vi "EventsRobotStuck.vi"(0 "our_robots":T3[](array[typedef]), 2 "Our_Robots frame":T1[](array[typedef]) {"height" format="%+4.3f"; "pixel_y" format="%+4.3f"; "pixel_x" format="%+4.3f"; "orientation" format="%+4.3f"; "y" format="%+4.3f"; "confidence" format="%4.3f"; "x" format="%+4.3f"}, 4 "FPS":dbl) -> (8 "Array":cluster{"ID":i32, "Relative error":dbl}[](array[cluster]))   [LabVIEW 2017]
uses:
  Core/AI Robot.ctl
  Intel/Functions Enum.ctl
  Intel/AttackerStates.ctl
  Path Planning/RRT/PathDests.ctl
  Path Planning/RRT/PathDest.ctl
  SSL Detection Robot.ctl
  <vilib>/Analysis/Matrix/Datatypes/RealMatrix.ctl
  <vilib>/Analysis/Matrix/NI_Matrix.lvlib
panel:
  out "Robot Stuck":bool
  out "empty?":bool
  out "Boolean":bool=TRUE
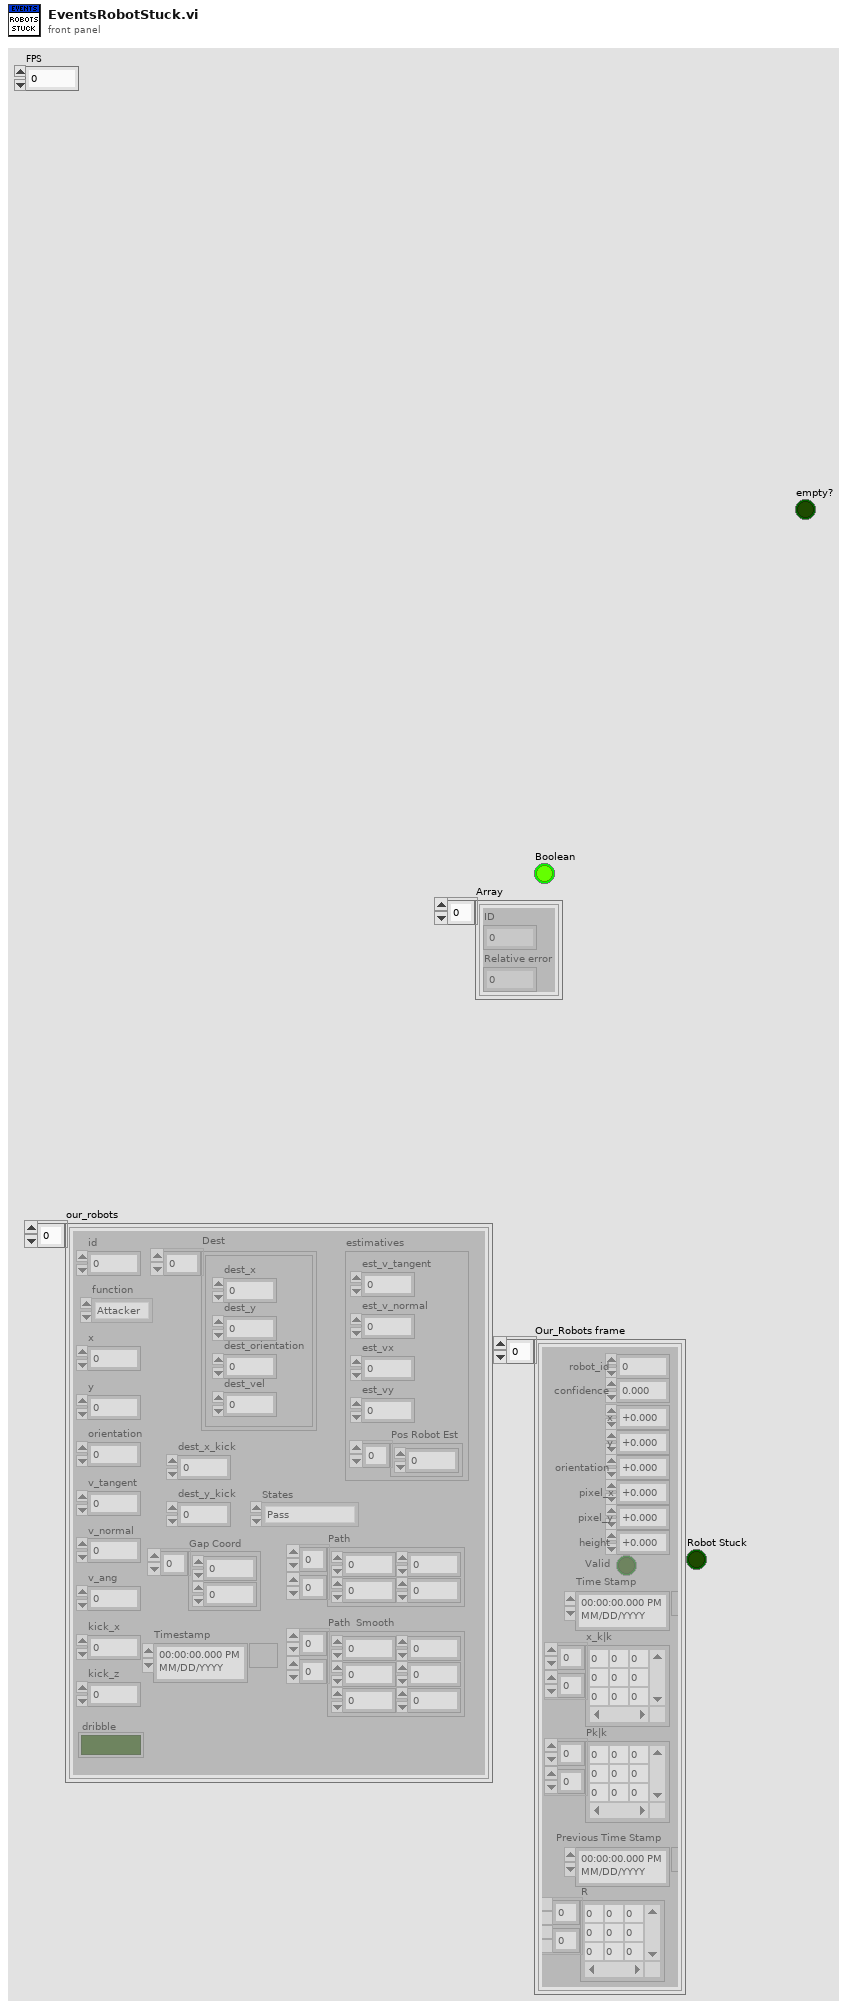
[diagram p1: front panel]
types:
  T1 = typedef "SSL Detection Robot.ctl" = cluster{"x":sgl, "robot_id":u32, "confidence":sgl, "y":sgl, "orientation":sgl, "pixel_x":sgl, "pixel_y":sgl, "height":sgl, "Valid":bool, "Time Stamp":timestamp, "x_k|k":T2, "Pk|k":T2, "Previous Time Stamp":timestamp, "R":T2}
  T2 = typedef "NI_Matrix.lvlib/RealMatrix.ctl" = dbl[][]
  T3 = typedef "AI Robot.ctl" = cluster{"id":u32, "function":T4, "x":dbl, "y":dbl, "orientation":dbl, "v_tangent":dbl, "v_normal":dbl, "v_ang":dbl, "kick_x":dbl, "kick_z":dbl, "dribble":bool, "Timestamp":timestamp, "estimatives":cluster{"est_v_tangent":dbl, "est_v_normal":dbl, "est_vx":dbl, "est_vy":dbl, "Pos Robot Est":dbl[]}, "dest_x_kick":dbl, "dest_y_kick":dbl, "Gap Coord":dbl[], "States":T5, "Path ":dbl[][], "Path  Smooth":dbl[][], "Dest":T6}
  T4 = typedef "Functions Enum.ctl" = enum16{"Attacker", "Goalie", "Defender", "Striker", "Goto 0", "Dummy", "Kicker", "ZigZag"}
  T5 = typedef "AttackerStates.ctl" = enum16{"Pass", "GoToTangent", "BallGetting", "GoToKick", ""}
  T6 = typedef "PathDests.ctl" = T7[]
  T7 = typedef "PathDest.ctl" = cluster{"dest_x":dbl, "dest_y":dbl, "dest_orientation":dbl, "dest_vel":dbl}
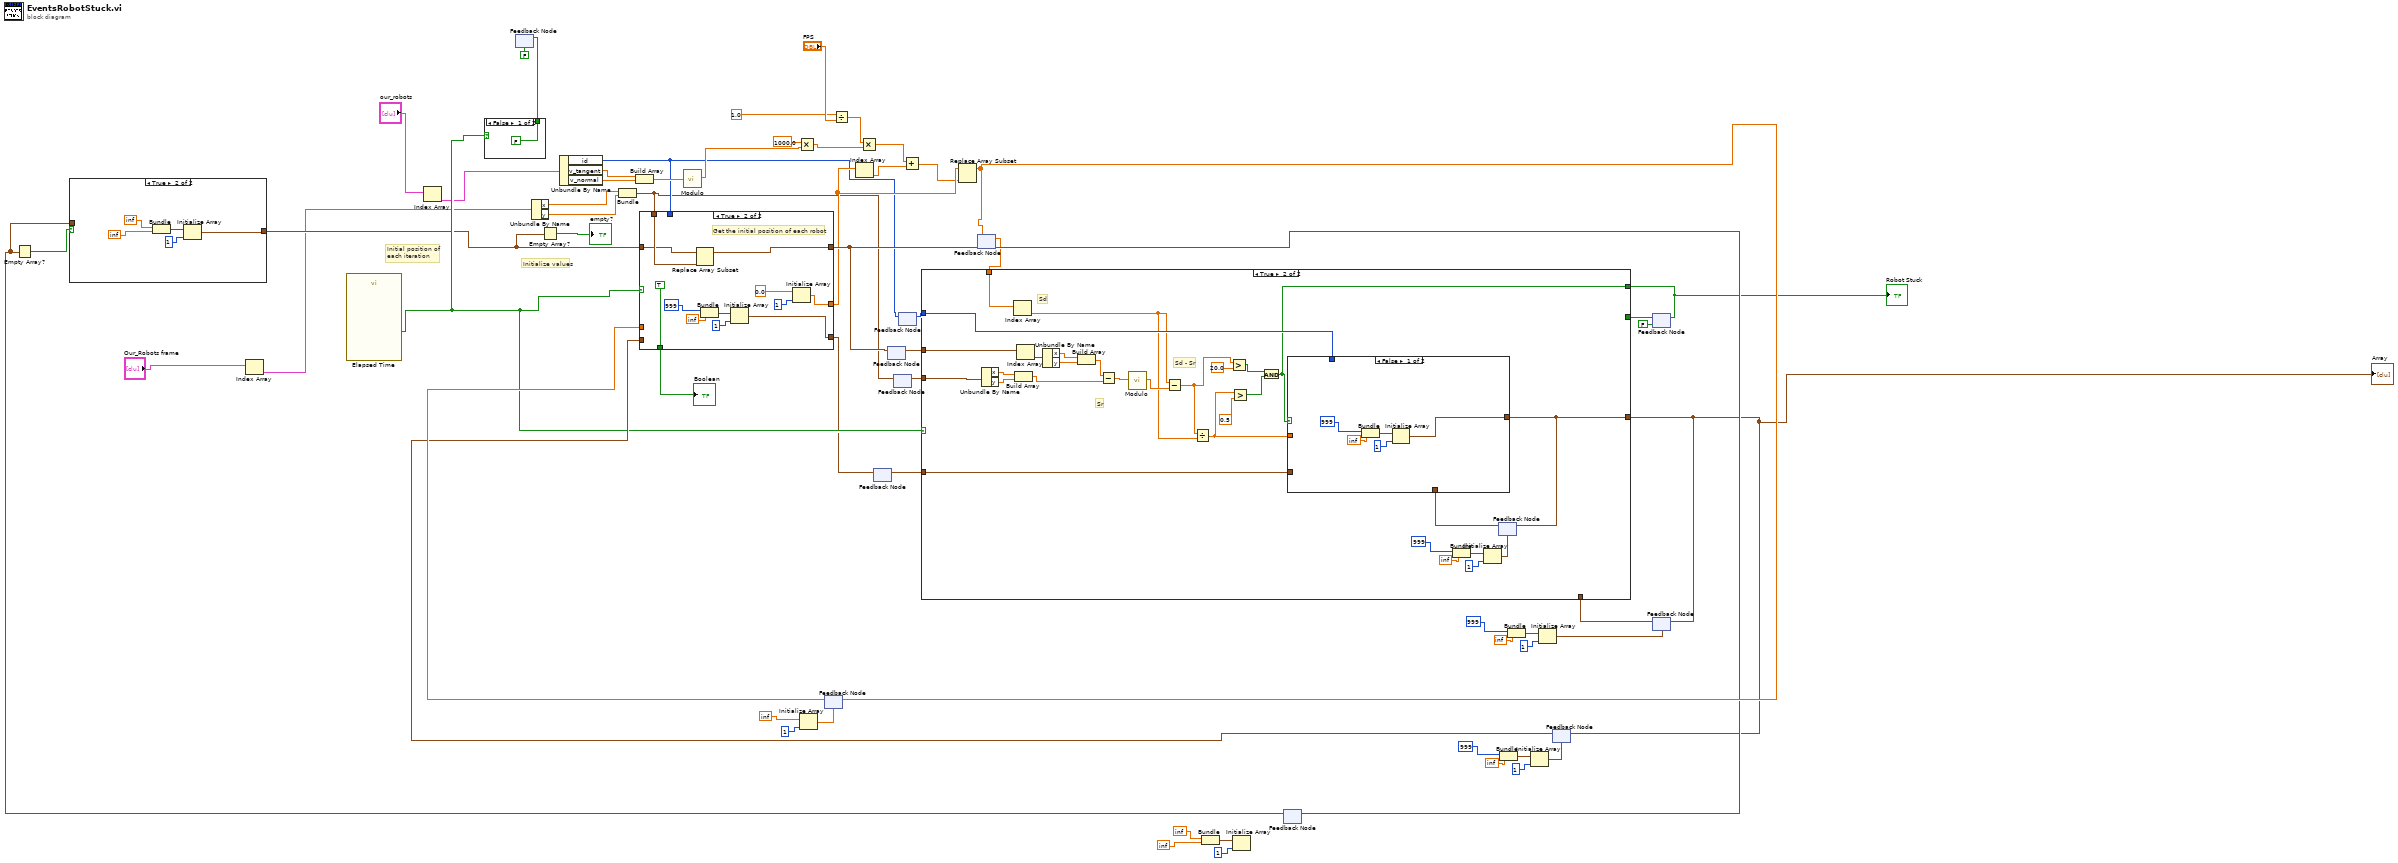
[diagram p0: block diagram]
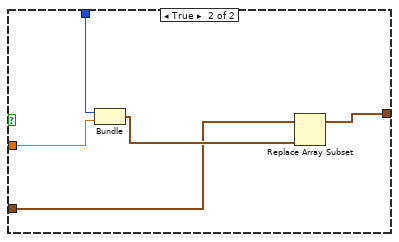
[diagram p3: hidden frame]
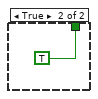
[diagram p4: hidden frame]
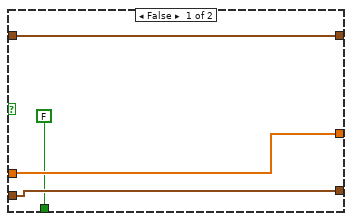
[diagram p5: hidden frame]
diagram:
  # "Initialize values"
  # "Initial position of\neach iteration"
  n1 = Index Array(array="Our_Robots frame") -> (element=w6:T1)  [unwired: 1 in]
  n2 = call "Elapsed Time"() -> ("Time has Elapsed"=w42:bool)  [unwired: 12 in, 7 out]
  n3 = Index Array(array="our_robots") -> (element=w3:T3)  [unwired: 1 in]
  n4 = case shown="False" w42 {
    tunnel: [FALSE TRUE] -> w50
    frame False {
    }
    frame True {
    }
  }
  n5 = feedback #1(FALSE) -> ()  [unwired: 1 in]
  n6 = feedback-in #1(w50) -> ()
  n7 = Unbundle By Name(w6) -> ("x"=w29:sgl, "y"=w28:sgl)
  n8 = Unbundle By Name(w3) -> ("id"=w11:u32, "v_tangent"=w38:dbl, "v_normal"=w37:dbl)
  n9 = Bundle("x"=w29, "y"=w28) -> (w8:cluster{"x":sgl, "y":sgl})  [unwired: 1 in]
  n10 = Build Array(w38, w37) -> (w36:dbl[])
  n11 = call "Modulo.vi"("2D vector"=w36) -> ("Modulo"=w27:dbl)  [unwired: 10 in]
  n12 = Multiply(x=1000.0, y=w27) -> (x*y=w25:dbl)
  n13 = Initialize Array(inf ("y"), 1 ("dimension size")) -> (w51:dbl[])
  n14 = feedback #2(w51) -> (w59:dbl[])
  n15 = Divide(x=1.0, y="FPS") -> (x/y=w33:dbl)
  n16 = Multiply(x=w33, y=w25) -> (x*y=w32:dbl)
  n17 = feedback #3() -> (w13:cluster{"ID":i32, "Relative error":dbl}[])  [unwired: 1 in]
  n18 = feedback #4() -> (w12:cluster{"x":sgl, "y":sgl}[])  [unwired: 1 in]
  n19 = feedback #5() -> (w7:cluster{"x":sgl, "y":sgl})  [unwired: 1 in]
  n20 = feedback-in #5(w8) -> ()
  n21 = feedback #6() -> (w10:u32)  [unwired: 1 in]
  n22 = feedback-in #6(w11) -> ()
  n23 = feedback #7() -> (w9:dbl[])  [unwired: 1 in]
  n24 = Bundle("x"=sgl inf, "y"=sgl inf) -> (w45:cluster{"x":sgl, "y":sgl})  [unwired: 1 in]
  n25 = Initialize Array(w45, 1 ("dimension size")) -> ()  [unwired: 1 out]
  n26 = feedback #8() -> (w39:cluster{"x":sgl, "y":sgl}[])  [unwired: 1 in]
  n27 = Empty Array?(array=w39) -> (empty?=w40:bool)
  n28 = case shown="True" w40 {
    tunnel: [w64 w65] -> w41
    tunnel: w39 -> [w64 _]
    frame False {
    }
    frame True {
      n29 = Bundle("x"=sgl inf, "y"=sgl inf) -> (w69:cluster{"x":sgl, "y":sgl})  [unwired: 1 in]
      n30 = Initialize Array(w69, 1 ("dimension size")) -> (w65:cluster{"x":sgl, "y":sgl}[])
    }
  }
  n31 = Empty Array?(array=w41) -> (empty?=→"empty?":bool)
  n32 = Bundle("dimension size"=999, "y"=inf) -> (w57:cluster{"dimension size":i32, "y":dbl})  [unwired: 1 in]
  n33 = Bundle("dimension size"=999, "y"=inf) -> (w18:cluster{"dimension size":i32, "y":dbl})  [unwired: 1 in]
  n34 = Initialize Array(w57, 1 ("dimension size")) -> (w55:cluster{"dimension size":i32, "y":dbl}[])
  n35 = Initialize Array(w18, 1 ("dimension size")) -> (w15:cluster{"dimension size":i32, "y":dbl}[])
  n36 = feedback #9(w55) -> (w48:cluster{"dimension size":i32, "y":dbl}[])
  n37 = case shown="True" w42 {
    tunnel: w59 -> [w73 _]
    tunnel: [w73 w81] -> w31
    tunnel: w8 -> [_ w84]
    tunnel: w11 -> [_ _]
    tunnel: [w72 w85] -> w47
    tunnel: w41 -> [w72 w83]
    tunnel: w48 -> [w71 _]
    tunnel: [w71 w77] -> w14
    tunnel: [FALSE TRUE] -> w24
    frame False {
    }
    frame True {
      # "Get the initial position of each robot"
      n38 = Replace Array Subset(array=w83, new element=w84) -> (w85:cluster{"x":sgl, "y":sgl}[])  [unwired: 1 in]
      n39 = Bundle("ID"=999, "Relative error"=inf) -> (w79:cluster{"ID":i32, "Relative error":dbl})  [unwired: 1 in]
      n40 = Initialize Array(w79, 1 ("dimension size")) -> (w77:cluster{"ID":i32, "Relative error":dbl}[])
      n41 = Initialize Array(0.0 ("element"), 1 ("dimension size")) -> (w81:dbl[])
    }
  }
  "Boolean" <- w24
  n42 = Index Array(array=w31) -> (element=w35:dbl)  [unwired: 1 in]
  n43 = feedback-in #3(w14) -> ()
  n44 = feedback-in #4(w47) -> ()
  n45 = Add(x=w32, y=w35) -> (x+y=w30:dbl)
  n46 = Replace Array Subset(array=w31, new element=w30) -> (w60:dbl[])  [unwired: 1 in]
  n47 = feedback-in #2(w60) -> ()
  n48 = feedback-in #7(w60) -> ()
  n49 = feedback-in #8(w47) -> ()
  n50 = feedback #10(FALSE) -> (w21:bool)
  n51 = feedback #11(w15) -> (w22:cluster{"dimension size":i32, "y":dbl}[])
  n52 = case shown="True" w42 {
    tunnel: w9 -> [_ w116]
    tunnel: w10 -> [_ w115]
    tunnel: w12 -> [_ w114]
    tunnel: w13 -> [_ w113]
    tunnel: w7 -> [_ w112]
    tunnel: [w87 w111] -> w1
    tunnel: [w86 w110] -> w2
    tunnel: w22 -> [w87 _]
    tunnel: w21 -> [w86 _]
    frame False {
    }
    frame True {
      # "Sr"
      # "Sd"
      # "Sd - Sr"
      n53 = Unbundle By Name(w112) -> ("x"=w105:sgl, "y"=w104:sgl)
      n54 = Index Array(array=w116) -> (element=w99:dbl)  [unwired: 1 in]
      n55 = Build Array(w105, w104) -> (w102:sgl[])
      n56 = Index Array(array=w114) -> (element=w109:cluster{"x":sgl, "y":sgl})  [unwired: 1 in]
      n57 = Unbundle By Name(w109) -> ("x"=w108:sgl, "y"=w107:sgl)
      n58 = Build Array(w108, w107) -> (w103:sgl[])
      n59 = Subtract(x=w103, y=w102) -> (x-y=w101:sgl[])
      n60 = call "Modulo.vi"("2D vector"=w101) -> ("Modulo"=w100:dbl)  [unwired: 10 in]
      n61 = Subtract(x=w99, y=w100) -> (x-y=w88:dbl)
      n62 = Divide(x=w88, y=w99) -> (x/y=w93:dbl)
      n63 = Greater?(x=w88, y=20.0) -> (0:w90:bool)
      n64 = Greater?(x=w93, y=0.5) -> (0:w91:bool)
      n65 = And(x=w90, y=w91) -> (x .and. y?=w110:bool)
      n66 = Bundle("dimension size"=999, "y"=inf) -> (w97:cluster{"dimension size":i32, "y":dbl})  [unwired: 1 in]
      n67 = Initialize Array(w97, 1 ("dimension size")) -> (w95:cluster{"dimension size":i32, "y":dbl}[])
      n68 = feedback #12(w95) -> (w106:cluster{"dimension size":i32, "y":dbl}[])
      n69 = case shown="False" w110 {
        tunnel: w115 -> [_ w122]
        tunnel: w93 -> [_ w126]
        tunnel: [w117 w125] -> w111
        tunnel: w106 -> [_ _]
        tunnel: w113 -> [_ w123]
        frame False {
          n70 = Bundle("dimension size"=999, "y"=inf) -> (w120:cluster{"dimension size":i32, "y":dbl})  [unwired: 1 in]
          n71 = Initialize Array(w120, 1 ("dimension size")) -> (w117:cluster{"dimension size":i32, "y":dbl}[])
        }
        frame True {
          n72 = Bundle("id"=w122, w126) -> (w124:cluster{"id":u32, dbl})  [unwired: 1 in]
          n73 = Replace Array Subset(array=w123, new element=w124) -> (w125:cluster{"ID":i32, "Relative error":dbl}[])  [unwired: 1 in]
        }
      }
      n74 = feedback-in #12(w111) -> ()
    }
  }
  "Robot Stuck" <- w2
  "Array" <- w1
  n75 = feedback-in #9(w1) -> ()
  n76 = feedback-in #10(w2) -> ()
  n77 = feedback-in #11(w1) -> ()
